vi "Example - Basic IPS-SA.vi"(0 "Connection Details":T6={"VISA resource name"="", "Comms Layer"=enum."Ethernet TCP/IP", "IP Address"="", "Serial Configuration"={"Baud Rate"=115200, "Parity"=0, "Data Bits"=8, "Stop Bits"=10, "Flow Control"=0}, "ISOBUS address"=-1} {"Serial Configuration"."Flow Control" items=["None", "XON/XOFF", "RTS/CTS", "XON/XOFF & RTS/CTS", "DTR/DSR", "XON/XOFF & DTR/DSR"]; "Serial Configuration"."Stop Bits" items=["1.0"=10, "2.0"=20]; "Serial Configuration"."Data Bits" items=["7"=7, "8"=8]; "Serial Configuration"."Parity" items=["None", "Odd", "Even"]; "Serial Configuration"."Baud Rate" items=["300"=300, "600"=600, "1200"=1200, "2400"=2400, "4800"=4800, "9600"=9600, "14400"=14400, "19200"=19200, "38400"=38400, "57600"=57600, "115200"=115200]}, 1 "Axis Group":string(combo)="GRPZ", 2 "ID Query (True)":bool, 3 "Clear Previous Connections (False)":bool, 4 "stop":bool, 6 "Ramp Controls":T8 {"Target Rate (T/min)" format="%_5g"; "Target Field (T)" format="%_5g"; "Target Rate (A/min)" format="%_5g"; "Target Current (A)" format="%_5g"}, 7 "Display Units":bool caption="AMP/TESLA", 8 "Magnet Controls":T9, 9 "SWITCH\nHEATER":bool, 11 "Sw Delay (s)":dbl=30.0 caption="Time Target (s)") -> (10 "System Time":string, 12 "Device Details":T2, 13 "SW HTR\nCONFIRM":bool, 14 "Output Current (A)":dbl format="%.4g", 15 "Magnet Current (A)":dbl format="%.4g", 16 "Output Voltage (V)":dbl format="%.4f", 17 "Current/Field (A/T)":dbl caption="Current Field Factor (A/T)" format="%#.4f", 19 "error out":errorcluster)   [LabVIEW 2013, in "Mercury iXX.lvlib"]
uses:
  Mercury iXX.lvlib
  Public/Libraries/Magnet/Signals/Read/Switch Heater Status (Read).vi
  Public/Libraries/Magnet.lvlib
  Public/Libraries/Magnet/Signals/Read/Current (Read).vi
  Public/Libraries/Magnet/Signals/Read/Persistant Current (Read).vi
  Public/Libraries/Magnet/Configuration/Set/PSU Action Status (Set).vi
  Public/Libraries/Magnet/Controls/PSU Actions.ctl
  Public/Libraries/Magnet/Controls/Switch Heater.ctl
  Public/Libraries/Temperature/Signals/Read/Temperature (Read).vi
  Public/Libraries/Temperature.lvlib
  Public/Libraries/Magnet/Configuration/Read/PSU Action Status (Read).vi
  Public/Libraries/Magnet/Signals/Set/Switch Heater No Check (Set).vi
  Public/Libraries/Magnet/Signals/Set/Target Field (Set).vi
  Public/Libraries/Magnet/Signals/Set/Target Current Rate (Set).vi
  Public/Libraries/Magnet/Signals/Set/Target Current (Set).vi
  Public/Libraries/Magnet/Signals/Set/Target Field Rate (Set).vi
  Public/Libraries/Level Meter/Signals/Read/Probe Level Helium (Read).vi
  Public/Libraries/Level Meter.lvlib
  Public/Libraries/Level Meter/Signals/Read/Probe Level Nitrogen (Read).vi
  Public/Libraries/Magnet/Configuration/Read/PSU Status (Read).vi
  Public/Libraries/System/Read/DateTime (Read).vi
  Public/Libraries/System.lvlib
  Public/Libraries/Pressure/Signals/Read/Current (Read).vi
  Public/Libraries/Pressure.lvlib
  Public/Libraries/System/Open/Open System.vi
  Public/Libraries/System/Read/Catalogue (Read).vi
  Public/Libraries/Level Meter/Open/Open Level Meter Device.vi
  Public/Libraries/Magnet/Open/Open Magnet Device.vi
  Public/Libraries/Magnet/Configuration/Read/Output Configuration (Read).vi
  Public/Libraries/Magnet/Configuration/Read/Current to Field Factor (Read).vi
  Public/Libraries/Temperature/Open/Open Temperature Device.vi
  Public/Libraries/Magnet/Signals/Read/Voltage (Read).vi
  Public/Controls/Comms Transport Layer.ctl
  Public/Controls/Serial Settings.ctl
  Public/Controls/ISOBus Address.ctl
  Public/Libraries/Magnet/Controls/Output Configuration.ctl
panel:
  out "Switch TS":timestamp
  out "Sentinel":bool
  in  "Tab Control":T1(tab)
  in  "Interval between messages (ms)":i16=100
  out "Number of Mag Units\nin the group":dbl
  out "Out Config 2":T7="PARA" caption="Output Configuration"
  out "Sys_time_stamp":timestamp
  out "Mode":string
  out "Nitrogen Level (%)":dbl format="%_4f"
  out "Helium Level (%)":dbl format="%_4f"
  out "Temperature (K)":dbl format="%_4f"
  out "Voltage (V)":dbl(knob) scale=-10.0..10.0
  out "Current (A)":dbl(knob) scale=-60.0..60.0
  out "Elapsed\nTime (s)":dbl caption="Elapsed Time (s)"
  out "Magnet Centre Field (T)":dbl format="%.4f"
  out "Output (T) (Field equivalent)":dbl format="%.4f"
  out "Status":string
  in  "Log file:":string="C:\\temp\\iPS_data.lvm"
  in  "Log Data?":bool
  in  "Plot Data?":bool
  out "Waveform Chart":T10(graph)
  # "Switch Controls"
  # "MercuryiPS-VI"
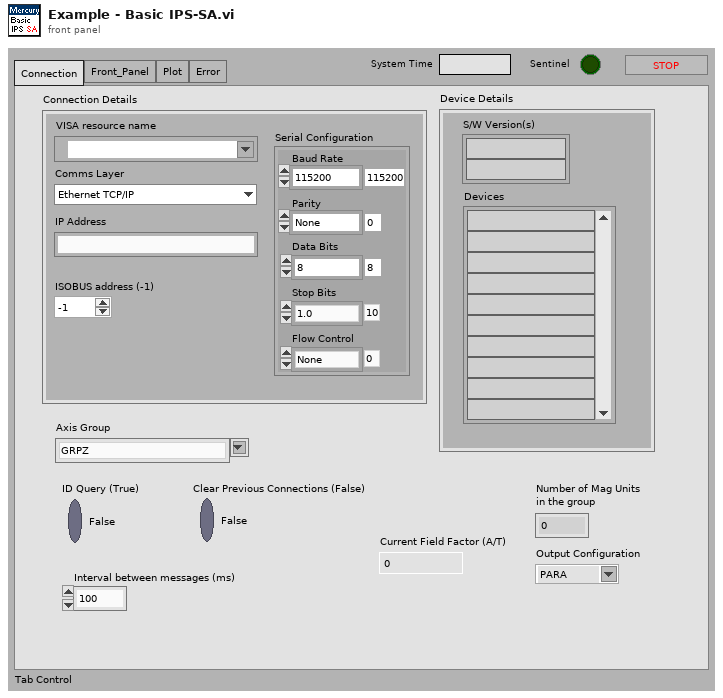
[diagram p1: front panel]
types:
  T1 = enum32{"Connection", "Front_Panel", "Plot", "Error"}
  T2 = cluster{"Devices":string[], "S/W Version(s)":string[]}
  T3 = typedef "Mercury iXX.lvlib/Comms Transport Layer.ctl" = enum16{"Ethernet TCP/IP", "USB", "ISOBus - RS-232", "GPIB"}
  T4 = typedef "Mercury iXX.lvlib/Serial Settings.ctl" = cluster{"Baud Rate":u32, "Parity":u16, "Data Bits":u16, "Stop Bits":u16, "Flow Control":u16}
  T5 = typedef "Mercury iXX.lvlib/ISOBus Address.ctl" = i32
  T6 = cluster{"VISA resource name":refnum<visa-resource-name>, "Comms Layer":T3, "IP Address":string, "Serial Configuration":T4, "ISOBUS address":T5}
  T7 = typedef "Mercury iXX.lvlib/Magnet.lvlib/Output Configuration.ctl" = string
  T8 = cluster{"Target Current (A)":dbl, "Target Rate (A/min)":dbl, "Target Field (T)":dbl, "Target Rate (T/min)":dbl}
  T9 = cluster{"CLAMP":bool, "HOLD":bool, "TO SET":bool, "TO ZERO":bool}
  T10 = cluster{"Current":dbl, "Persistant Current":dbl, "Voltage":dbl, "Temperature":dbl}
  T11 = typedef "Mercury iXX.lvlib/Mercury Reference.ctl" = cluster{"Comms":refnum<visa-resource-name>, "Device ID":string[], "Comms Layer":T3, "Command":string, "Query reference":T12}
  T12 = typedef "Mercury iXX.lvlib/Query Dynamic Reference.ctl" = refnum<vi>
  T13 = typedef "Mercury iXX.lvlib/Magnet.lvlib/PSU Actions.ctl" = string
  T14 = typedef "Mercury iXX.lvlib/Magnet.lvlib/Switch Heater.ctl" = string
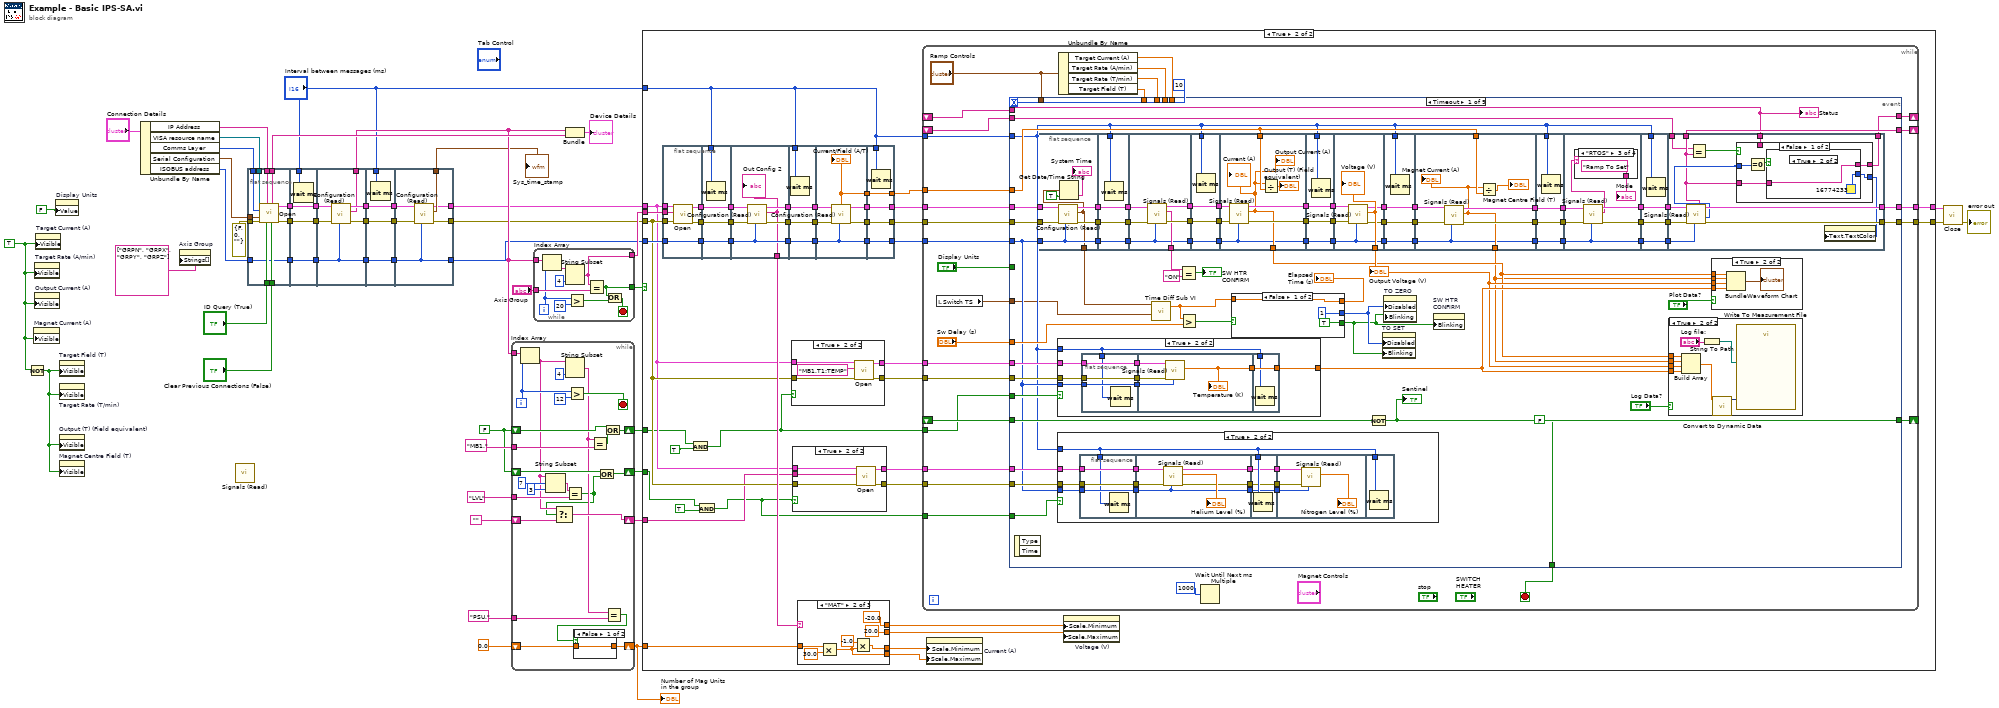
[diagram p0: block diagram]
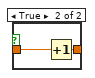
[diagram p2: hidden frame]
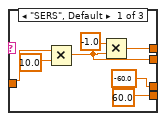
[diagram p6: hidden frame]
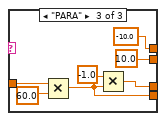
[diagram p7: hidden frame]
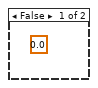
[diagram p8: hidden frame]
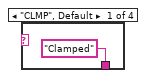
[diagram p9: hidden frame]
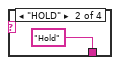
[diagram p10: hidden frame]
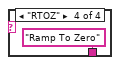
[diagram p11: hidden frame]
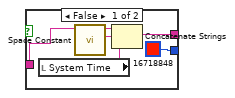
[diagram p12: hidden frame]
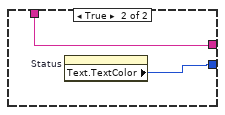
[diagram p13: hidden frame]
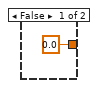
[diagram p14: hidden frame]
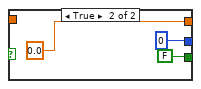
[diagram p17: hidden frame]
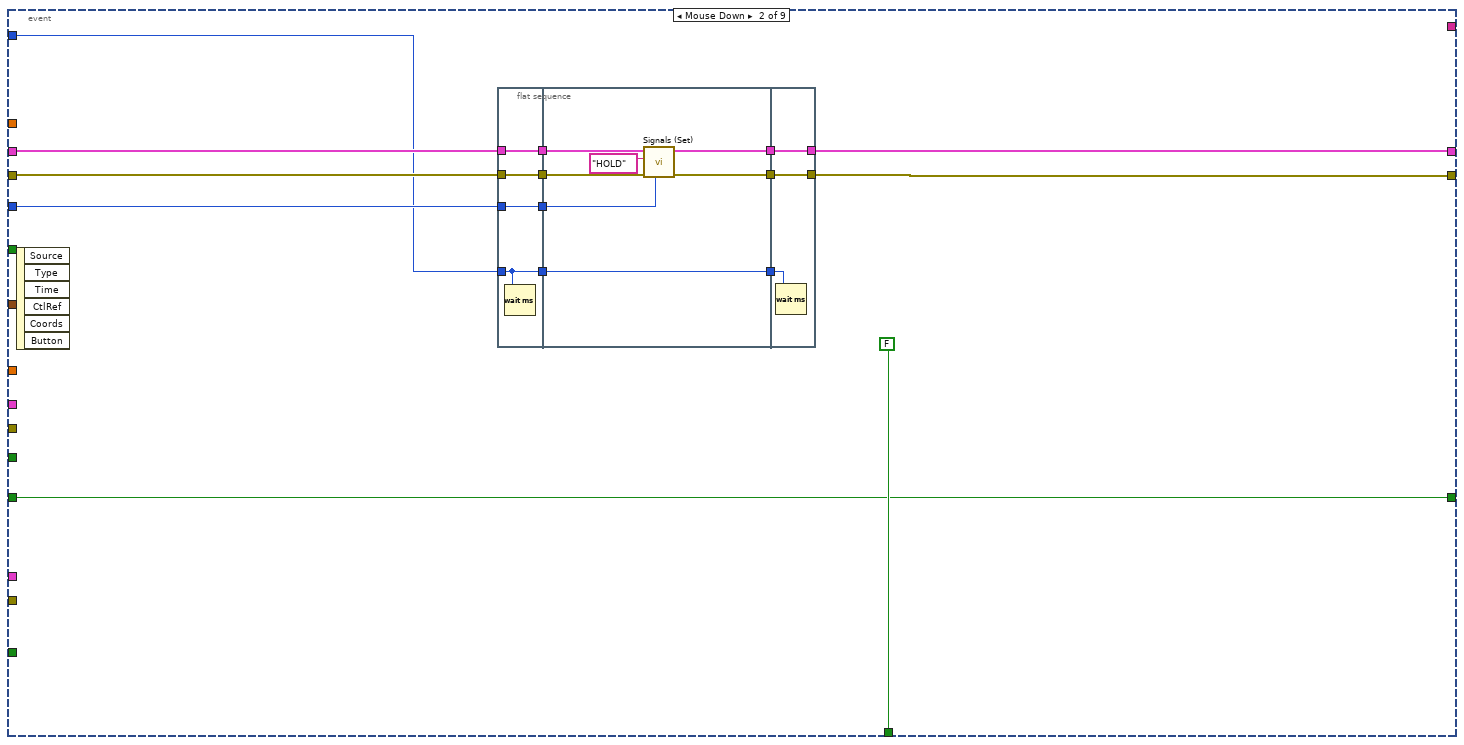
[diagram p18: hidden frame]
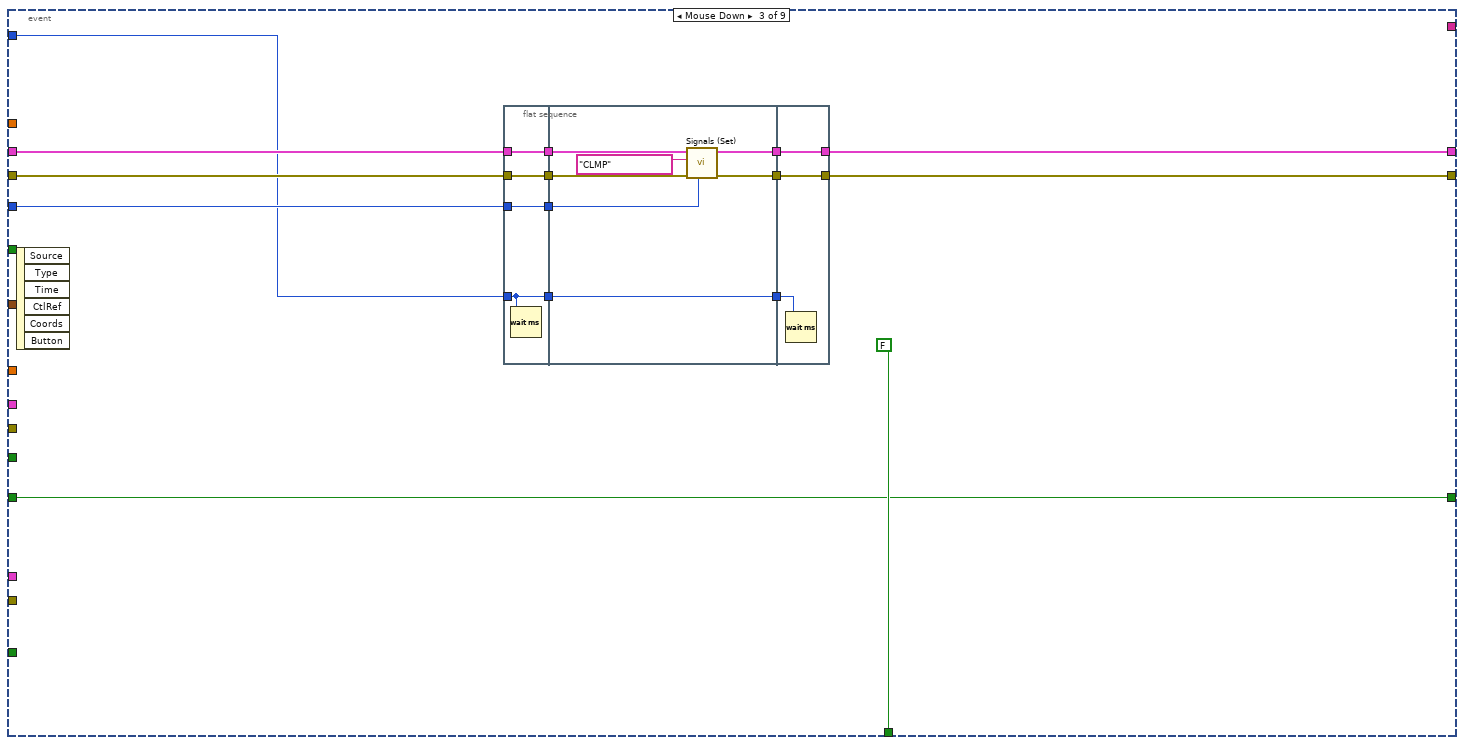
[diagram p19: hidden frame]
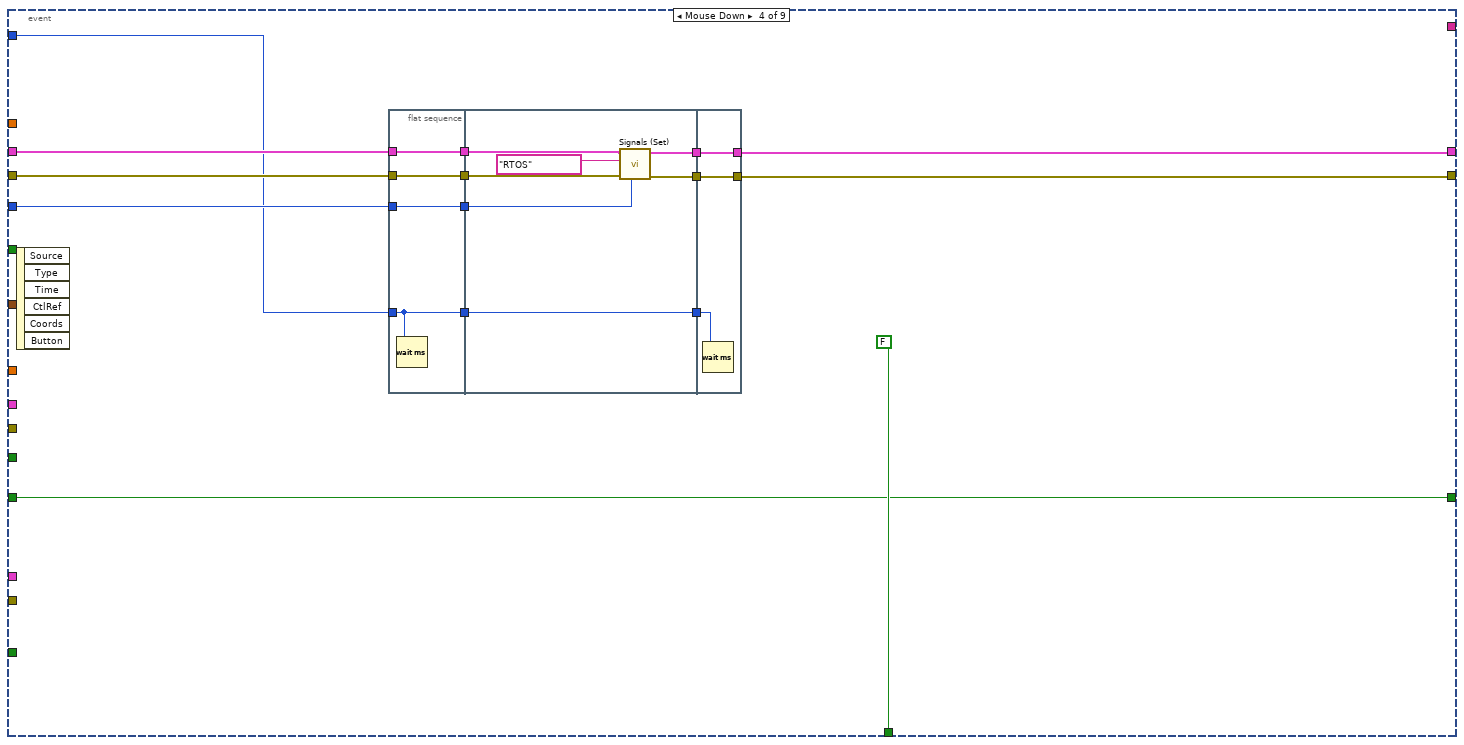
[diagram p20: hidden frame]
diagram:
  w13 = FALSE
  w35 = TRUE ("Visible")
  n1 = Not(x=w35) -> (.not. x?=w34:bool)
  n2 = property on="Magnet Current (A)" class="DigNum (strict)"("Visible"=w35) -> ()  [unwired: 2 in, 2 out]
  n3 = property on="Target Rate (A/min)" class="DigNum (strict)"("Visible"=w35) -> ()  [unwired: 2 in, 2 out]
  n4 = property on="Output Current (A)" class="DigNum (strict)"("Visible"=w35) -> ()  [unwired: 2 in, 2 out]
  n5 = property on="Target Current (A)" class="DigNum (strict)"("Visible"=w35) -> ()  [unwired: 2 in, 2 out]
  n6 = property on="Display Units" class="Bool (strict)"("Value"=FALSE ("AMP/TESLA")) -> ()  [unwired: 2 in, 2 out]
  n7 = property on="Target Field (T)" class="DigNum (strict)"("Visible"=w34) -> ()  [unwired: 2 in, 2 out]
  n8 = property on="Target Rate (T/min)" class="DigNum (strict)"("Visible"=w34) -> ()  [unwired: 2 in, 2 out]
  n9 = property on="Output (T) (Field equivalent)" class="DigNum (strict)"("Visible"=w34) -> ()  [unwired: 2 in, 2 out]
  n10 = property on="Magnet Centre Field (T)" class="DigNum (strict)"("Visible"=w34) -> ()  [unwired: 2 in, 2 out]
  n11 = Unbundle By Name("Connection Details") -> ("IP Address"=w31:string, "VISA resource name"=w30:refnum<visa-resource-name>, "Comms Layer"=w29:T3, "Serial Configuration"=w32:T4, "ISOBUS address"=w20:T5)
  n12 = property on="Axis Group" class="CmbBox"("Strings[]"=string[] ["GRPN", "GRPX", "GRPY", "GRPZ"]) -> ()  [unwired: 2 in, 2 out]
  n13 = call-poly "Signals (Read).vi"() -> ()  [unwired: 7 in, 5 out]
  n14 = flat-sequence {
    tunnel: errorcluster {"status"=FALSE, "code"=0, "source"=""} ("error in (no error)") -> [w60]
    tunnel: "ID Query (True)" -> [w59]
    tunnel: "Clear Previous Connections (False)" -> [w58]
    tunnel: w32 -> [w55]
    tunnel: w31 -> [w54]
    tunnel: w30 -> [w53]
    tunnel: w29 -> [w52]
    tunnel: [w51] -> w27
    tunnel: [w57] -> w24
    tunnel: [w56] -> w23
    tunnel: w20 -> [w50]
    tunnel: [w50] -> w19
    tunnel: w24 -> [w64]
    tunnel: w23 -> [w63]
    tunnel: [w64] -> w22
    tunnel: [w63] -> w21
    tunnel: w19 -> [w62]
    tunnel: [w62] -> w18
    tunnel: "Interval between messages (ms)" -> [w61]
    tunnel: w22 -> [w69]
    tunnel: w21 -> [w68]
    tunnel: w18 -> [w70]
    tunnel: [w70] -> w17
    tunnel: [w67] -> w16
    tunnel: [w66] -> w15
    tunnel: [w65] -> w6
    tunnel: w17 -> [w74]
    tunnel: w16 -> [w73]
    tunnel: w15 -> [w72]
    tunnel: "Interval between messages (ms)" -> [w71]
    tunnel: [w74] -> w9
    tunnel: [w73] -> w8
    tunnel: [w72] -> w7
    tunnel: w9 -> [w78]
    tunnel: w8 -> [w79]
    tunnel: w7 -> [w80]
    tunnel: [w77] -> w1
    tunnel: [w78] -> w5
    tunnel: [w76] -> w3
    tunnel: [w75] -> w2
    frame #0 {
      n15 = call-poly "Open.vi"("Clear Previous Connections (False)"=w58, "ID Query (True)"=w59, "IP Address"=w54, "error in (no error)"=w60, "Serial Configuration"=w55, "Comms Layer"=w52, "VISA resource name"=w53) -> ("error out"=w56:errorcluster, "Mercury Reference Out"=w57:T11, "S/W Version(s)"=w51:string[])  [unwired: 2 out]
    }
    frame #1 {
      n16 = Wait (ms)(milliseconds to wait=w61) -> ()  [unwired: 1 out]
    }
    frame #2 {
      n17 = call-poly "Configuration (Read).vi"("ISOBUS address"=w70, "error in"=w68, "Mercury Reference In"=w69) -> ("error out"=w67:errorcluster, "Devices"=w65:string[], "Mercury Reference Out"=w66:T11)  [unwired: 6 out]
    }
    frame #3 {
      n18 = Wait (ms)(milliseconds to wait=w71) -> ()  [unwired: 1 out]
    }
    frame #4 {
      n19 = call-poly "Configuration (Read).vi"("ISOBUS address"=w78, "error in"=w79, "Mercury Reference In"=w80) -> ("error out"=w75:errorcluster, "time stamp"=w77:timestamp, "Mercury Reference Out"=w76:T11)  [unwired: 6 out]
    }
  }
  n20 = while {
    shift-right: [w101] -> w37
    shift-left: 0.0 -> [w100]
    tunnel: "PSU." -> [w97]
    tunnel: w6 -> [w96]
    shift-right: [w93] -> w25
    shift-left: w13 -> [w92]
    tunnel: "MB1." -> [w94]
    tunnel: "LVL" -> [w88]
    shift-right: [w86] -> w12
    shift-left: w13 -> [w87]
    shift-right: [w84] -> w10
    shift-left: "" -> [w85]
    i -> [w102]
    stop <- w98 stop-if-true
    n21 = Index Array(array=w96, index=w102) -> (element=w82:string)
    n22 = String Subset(string=w82, offset (0)=7, length (rest)=3 ("length (rest)")) -> (substring=w89:string)
    n23 = String Subset(string=w82, length (rest)=4 ("length (rest)")) -> (substring=w83:string)  [unwired: 1 out]
    n24 = Equal?(x=w89, y=w88) -> (x = y?=w81:bool)
    n25 = Select(t=w82, s=w81, f=w85) -> (s? t:f=w84:string)
    n26 = Greater?(x=w102, y=12) -> (0:w98:bool)
    n27 = Equal?(x=w83, y=w94) -> (x = y?=w95:bool)
    n28 = Or(x=w87, y=w81) -> (x .or. y?=w86:bool)
    n29 = Or(x=w92, y=w95) -> (x .or. y?=w93:bool)
    n30 = Equal?(x=w83, y=w97) -> (x = y?=w99:bool)
    n31 = case shown="False" w99 {
      tunnel: [w105 w107] -> w101
      tunnel: w100 -> [w105 w106]
      frame False {
      }
      frame True {
        n32 = Increment(x=w106) -> (x+1=w107:dbl)
      }
    }
  }
  "Number of Mag Units\nin the group" <- w37
  n33 = while {
    tunnel: w6 -> [w117]
    tunnel: [w108] -> w45
    tunnel: "Axis Group" -> [w114]
    tunnel: [w109] -> w46
    i -> [w112]
    stop <- w111 stop-if-true
    n34 = Index Array(array=w117, index=w112) -> (element=w115:string)
    n35 = String Subset(string=w115, length (rest)=4 ("length (rest)")) -> (substring=w108:string)  [unwired: 1 out]
    n36 = Greater?(x=w112, y=20) -> (0:w110:bool)
    n37 = Equal?(x=w108, y=w114) -> (x = y?=w109:bool)
    n38 = Or(x=w109, y=w110) -> (x .or. y?=w111:bool)
  }
  n39 = Bundle("Devices"=w6, "S/W Version(s)"=w27) -> (→"Device Details":T2)  [unwired: 1 out]
  n40 = case shown="True" w46 {
    tunnel: w3 -> [w119 w129]
    tunnel: w45 -> [_ w163]
    tunnel: w5 -> [_ w153]
    tunnel: [w119 w162] -> w44
    tunnel: [w118 w161] -> w43
    tunnel: w37 -> [_ w160]
    tunnel: w2 -> [w118 w130]
    tunnel: w25 -> [_ w125]
    tunnel: "Interval between messages (ms)" -> [_ w131]
    tunnel: w12 -> [_ w123]
    tunnel: w10 -> [_ w128]
    frame False {
    }
    frame True {
      n41 = flat-sequence {
        tunnel: w163 -> [w176]
        tunnel: w130 -> [w173]
        tunnel: w129 -> [w172]
        tunnel: w153 -> [w171]
        tunnel: [w175] -> w152
        tunnel: [w174] -> w151
        tunnel: [w171] -> w150
        tunnel: w152 -> [w180]
        tunnel: w151 -> [w179]
        tunnel: w150 -> [w178]
        tunnel: [w180] -> w149
        tunnel: [w179] -> w148
        tunnel: [w178] -> w147
        tunnel: w131 -> [w177]
        tunnel: w149 -> [w186]
        tunnel: w148 -> [w185]
        tunnel: w147 -> [w184]
        tunnel: [w181] -> w146
        tunnel: [w184] -> w145
        tunnel: [w183] -> w144
        tunnel: [w182] -> w143
        tunnel: w145 -> [w190]
        tunnel: w144 -> [w189]
        tunnel: w143 -> [w188]
        tunnel: [w190] -> w142
        tunnel: [w189] -> w141
        tunnel: [w188] -> w140
        tunnel: w131 -> [w187]
        tunnel: w142 -> [w192]
        tunnel: w141 -> [w196]
        tunnel: w140 -> [w195]
        tunnel: [w192] -> w139
        tunnel: [w194] -> w138
        tunnel: [w193] -> w137
        tunnel: [w191] -> w136
        tunnel: [w198] -> w135
        tunnel: [w199] -> w133
        tunnel: [w200] -> w134
        tunnel: [w201] -> w132
        tunnel: w139 -> [w201]
        tunnel: w138 -> [w200]
        tunnel: w137 -> [w199]
        tunnel: w136 -> [w198]
        tunnel: w131 -> [w197]
        frame #0 {
          n42 = call-poly "Open.vi"("error in (no error)"=w173, "Device Identifier"=w176, "Mercury Reference In"=w172) -> ("error out"=w174:errorcluster, "Mercury Reference Out"=w175:T11)  [unwired: 7 out]
        }
        frame #1 {
          n43 = Wait (ms)(milliseconds to wait=w177) -> ()  [unwired: 1 out]
        }
        frame #2 {
          n44 = call-poly "Configuration (Read).vi"("ISOBUS address"=w184, "error in"=w185, "Mercury Reference In"=w186) -> ("error out"=w182:errorcluster, "Out Config"=w181:T7, "Mercury Reference Out"=w183:T11)  [unwired: 6 out]
          "Out Config 2" <- w181
        }
        frame #3 {
          n45 = Wait (ms)(milliseconds to wait=w187) -> ()  [unwired: 1 out]
        }
        frame #4 {
          n46 = call-poly "Configuration (Read).vi"("ISOBUS address"=w192, "error in"=w195, "Mercury Reference In"=w196) -> ("error out"=w193:errorcluster, "AtoB"=w191:dbl, "Mercury Reference Out"=w194:T11)  [unwired: 6 out]
          "Current/Field (A/T)" <- w191
        }
        frame #5 {
          n47 = Wait (ms)(milliseconds to wait=w197) -> ()  [unwired: 1 out]
        }
      }
      n48 = And(x=w125, y=TRUE) -> (x .and. y?=w124:bool)
      n49 = And(x=w123, y=TRUE) -> (x .and. y?=w122:bool)
      n50 = case shown="True" w124 {
        tunnel: w130 -> [w202 w207]
        tunnel: w129 -> [w203 w206]
        tunnel: [w203 w205] -> w155
        tunnel: [w202 w204] -> w154
        frame False {
        }
        frame True {
          n51 = call-poly "Open.vi"("error in (no error)"=w207, "Device Identifier"="MB1.T1:TEMP", "Mercury Reference In"=w206) -> ("error out"=w204:errorcluster, "Mercury Reference Out"=w205:T11)  [unwired: 7 out]
        }
      }
      n52 = case shown="True" w122 {
        tunnel: w130 -> [w164 w170]
        tunnel: w129 -> [w165 w169]
        tunnel: [w165 w168] -> w127
        tunnel: [w164 w167] -> w126
        tunnel: w128 -> [_ w166]
        frame False {
        }
        frame True {
          n53 = call-poly "Open.vi"("error in (no error)"=w170, "Device Identifier"=w166, "Mercury Reference In"=w169) -> ("error out"=w167:errorcluster, "Mercury Reference Out"=w168:T11)  [unwired: 7 out]
        }
      }
      n54 = case shown="\"MAT\"" w146 {
        tunnel: w160 -> [w213 w220 w229]
        tunnel: [60.0 ("y") w219 w226] -> w158
        tunnel: [-60.0 ("y") w218 w225] -> w159
        tunnel: [w212 -20.0 ("y") -10.0 ("y")] -> w157
        tunnel: [w211 20.0 ("y") 10.0 ("y")] -> w156
        frame "SERS", Default {
          n55 = Multiply(x=w213, y=10.0) -> (x*y=w211:dbl)
          n56 = Multiply(x=-1.0, y=w211) -> (x*y=w212:dbl)
        }
        frame "MAT" {
          n57 = Multiply(x=w220, y=30.0) -> (x*y=w219:dbl)
          n58 = Multiply(x=-1.0, y=w219) -> (x*y=w218:dbl)
        }
        frame "PARA" {
          n59 = Multiply(x=w229, y=60.0) -> (x*y=w226:dbl)
          n60 = Multiply(x=-1.0, y=w226) -> (x*y=w225:dbl)
        }
      }
      n61 = while {
        tunnel: w134 -> [w257]
        tunnel: w133 -> [w256]
        shift-right: [w254] -> _
        shift-left: _ -> [w255]
        tunnel: [w252] -> w162
        tunnel: [w251] -> w161
        tunnel: w135 -> [w249]
        tunnel: w155 -> [w242]
        tunnel: w154 -> [w241]
        tunnel: w124 -> [w243]
        tunnel: w132 -> [w240]
        tunnel: w131 -> [w239]
        tunnel: w127 -> [w238]
        tunnel: w126 -> [w237]
        tunnel: w122 -> [w236]
        shift-right: [w235] -> _
        shift-left: _ -> [w234]
        shift-right: [w233] -> _
        shift-left: _ -> [w232]
        stop <- w253 stop-if-true
        n62 = local read "Switch TS"() -> (w231:timestamp)
        n63 = Unbundle By Name("Ramp Controls") -> ("Target Current (A)"=w246:dbl, "Target Rate (A/min)"=w247:dbl, "Target Rate (T/min)"=w245:dbl, "Target Field (T)"=w244:dbl)
        n64 = event shown="[0] Timeout" {
          selector: _ -> [_ _ _ _ _ _ _ _ _]
          dyn-events: _ -> [_ _ _ _ _ _ _ _ _]
          timeout: 10 -> [_ _ _ _ _ _ _ _ _]
          tunnel: w257 -> [w316 w514 w544 w573 w602 w639 w754 w874 w877]
          tunnel: w256 -> [w315 w515 w543 w572 w601 w638 w753 w873 w888]
          tunnel: w255 -> [w330 w510 w539 w568 w597 w643 w749 w875 _]
          tunnel: [w329 w510 w539 w568 w597 w643 w749 w875 _] -> w254
          tunnel: [w290 w513 w542 w571 w600 w642 w752 w874 w877] -> w252
          tunnel: [w289 w512 w541 w570 w599 w641 w751 w873 w880] -> w251
          tunnel: [FALSE FALSE FALSE FALSE FALSE FALSE FALSE TRUE _] -> w253
          tunnel: "Sw Delay (s)" -> [w327 _ _ _ _ _ _ _ _]
          tunnel: w249 -> [w278 _ _ _ _ _ w740 _ _]
          tunnel: "Display Units" -> [_ _ _ _ _ _ w748 _ w879]
          tunnel: w247 -> [_ _ _ _ _ _ w747 _ _]
          tunnel: w246 -> [_ _ _ _ _ _ w746 _ _]
          tunnel: w245 -> [_ _ _ _ _ _ w745 _ _]
          tunnel: w244 -> [_ _ _ _ _ _ w744 _ _]
          tunnel: w243 -> [w320 _ _ _ _ _ _ _ _]
          tunnel: w242 -> [w319 _ _ _ _ _ _ _ _]
          tunnel: w241 -> [w318 _ _ _ _ _ _ _ _]
          tunnel: w240 -> [w273 w509 w538 w567 w596 w637 w743 _ _]
          tunnel: w239 -> [w272 w501 w530 w559 w588 w617 w742 _ _]
          tunnel: w238 -> [w275 _ _ _ _ _ _ _ _]
          tunnel: w237 -> [w274 _ _ _ _ _ _ _ _]
          tunnel: w236 -> [w271 _ _ _ _ _ _ _ _]
          tunnel: [w266 _ _ _ _ _ _ _ _] -> w235
          tunnel: w234 -> [w265 _ _ _ _ _ _ _ _]
          tunnel: [w264 _ _ _ _ _ _ _ _] -> w233
          tunnel: w232 -> [w260 _ _ _ _ _ _ _ _]
          tunnel: w231 -> [w262 _ _ _ _ _ _ _ _]
          tunnel: "Ramp Controls" -> [_ _ _ _ _ _ w741 _ _]
          event Timeout {
            n65 = event-data() -> ()  [unwired: 3 out]
            n66 = flat-sequence {
              tunnel: [w367] -> w263
              tunnel: w316 -> [w372]
              tunnel: w315 -> [w371]
              tunnel: [w370] -> w314
              tunnel: [w369] -> w313
              tunnel: w273 -> [w368]
              tunnel: [w368] -> w287
              tunnel: w314 -> [w376]
              tunnel: w313 -> [w375]
              tunnel: [w376] -> w312
              tunnel: [w375] -> w311
              tunnel: [w374] -> w288
              tunnel: w287 -> [w374]
              tunnel: w272 -> [w373]
              tunnel: w312 -> [w381]
              tunnel: w311 -> [w382]
              tunnel: [w378] -> w310
              tunnel: [w380] -> w309
              tunnel: [w379] -> w308
              tunnel: w288 -> [w377]
              tunnel: [w377] -> w285
              tunnel: w309 -> [w386]
              tunnel: w308 -> [w385]
              tunnel: [w386] -> w307
              tunnel: [w385] -> w306
              tunnel: [w384] -> w286
              tunnel: w285 -> [w384]
              tunnel: w272 -> [w383]
              tunnel: w307 -> [w394]
              tunnel: w306 -> [w393]
              tunnel: w278 -> [w391]
              tunnel: [w390] -> w305
              tunnel: [w389] -> w304
              tunnel: [w388] -> w300
              tunnel: w286 -> [w387]
              tunnel: [w387] -> w283
              tunnel: w305 -> [w398]
              tunnel: w304 -> [w397]
              tunnel: [w398] -> w303
              tunnel: [w397] -> w302
              tunnel: [w396] -> w284
              tunnel: w283 -> [w396]
              tunnel: w272 -> [w395]
              tunnel: w303 -> [w404]
              tunnel: w302 -> [w403]
              tunnel: [w402] -> w301
              tunnel: [w401] -> w299
              tunnel: [w400] -> w298
              tunnel: w284 -> [w399]
              tunnel: [w399] -> w281
              tunnel: w299 -> [w408]
              tunnel: w298 -> [w407]
              tunnel: [w408] -> w297
              tunnel: [w407] -> w296
              tunnel: [w406] -> w282
              tunnel: w281 -> [w406]
              tunnel: w272 -> [w405]
              tunnel: w297 -> [w416]
              tunnel: w296 -> [w415]
              tunnel: w278 -> [w411]
              tunnel: [w410] -> w295
              tunnel: [w414] -> w294
              tunnel: [w413] -> w293
              tunnel: w282 -> [w409]
              tunnel: [w409] -> w279
              tunnel: w294 -> [w420]
              tunnel: w293 -> [w419]
              tunnel: [w420] -> w292
              tunnel: [w419] -> w291
              tunnel: [w418] -> w280
              tunnel: w279 -> [w418]
              tunnel: w272 -> [w417]
              tunnel: w292 -> [w426]
              tunnel: w291 -> [w427]
              tunnel: w280 -> [w423]
              tunnel: [w425] -> w277
              tunnel: [w424] -> w276
              tunnel: [w423] -> w267
              tunnel: w277 -> [w435]
              tunnel: w276 -> [w434]
              tunnel: w272 -> [w433]
              tunnel: [w435] -> w270
              tunnel: [w434] -> w269
              tunnel: [w432] -> w268
              tunnel: w267 -> [w432]
              tunnel: [w444] -> w289
              tunnel: [w445] -> w290
              tunnel: w270 -> [w446]
              tunnel: w269 -> [w447]
              tunnel: w268 -> [w443]
              tunnel: [w439] -> w266
              tunnel: w265 -> [w438]
              tunnel: [w437] -> w264
              tunnel: w260 -> [w436]
              frame #0 {
                n67 = call-poly "Configuration (Read).vi"("ISOBUS address"=w368, "error in"=w371, "Mercury Reference In"=w372) -> ("error out"=w369:errorcluster, "time stamp"=w367:timestamp, "Mercury Reference Out"=w370:T11)  [unwired: 6 out]
                n68 = Get Date/Time String(seconds (now)=w367, want seconds? (F)=TRUE) -> (time string=→"System Time":string)  [unwired: 1 in, 1 out]
              }
              frame #1 {
                n69 = Wait (ms)(milliseconds to wait=w373) -> ()  [unwired: 1 out]
              }
              frame #2 {
                n70 = call-poly "Signals (Read).vi"("ISOBUS address"=w377, "error in"=w382, "Mercury Reference In"=w381) -> ("error out"=w379:errorcluster, "Switch Heater Status"=w378:string, "Mercury Reference Out"=w380:T11)  [unwired: 6 out]
              }
              frame #3 {
                n71 = Wait (ms)(milliseconds to wait=w383) -> ()  [unwired: 1 out]
              }
              frame #4 {
                n72 = call-poly "Signals (Read).vi"("ISOBUS address"=w387, "error in"=w393, "Mercury Reference In"=w394) -> ("error out"=w389:errorcluster, "Current"=w388:dbl, "Mercury Reference Out"=w390:T11)  [unwired: 6 out]
                "Current (A)" <- w388
                "Output Current (A)" <- w388
                n73 = Divide(x=w388, y=w391) -> (x/y=→"Output (T) (Field equivalent)":dbl)
              }
              frame #5 {
                n74 = Wait (ms)(milliseconds to wait=w395) -> ()  [unwired: 1 out]
              }
              frame #6 {
                n75 = call-poly "Signals (Read).vi"("ISOBUS address"=w399, "error in"=w403, "Mercury Reference In"=w404) -> ("error out"=w400:errorcluster, "Voltage"=w402:dbl, "Mercury Reference Out"=w401:T11)  [unwired: 6 out]
                "Voltage (V)" <- w402
              }
              frame #7 {
                n76 = Wait (ms)(milliseconds to wait=w405) -> ()  [unwired: 1 out]
              }
              frame #8 {
                n77 = call-poly "Signals (Read).vi"("ISOBUS address"=w409, "error in"=w415, "Mercury Reference In"=w416) -> ("error out"=w414:errorcluster, "Persistant Current"=w410:dbl, "Mercury Reference Out"=w413:T11)  [unwired: 6 out]
                "Magnet Current (A)" <- w410
                n78 = Divide(x=w410, y=w411) -> (x/y=→"Magnet Centre Field (T)":dbl)
              }
              frame #9 {
                n79 = Wait (ms)(milliseconds to wait=w417) -> ()  [unwired: 1 out]
              }
              frame #10 {
                n80 = call-poly "Signals (Read).vi"("ISOBUS address"=w423, "error in"=w426, "Mercury Reference In"=w427) -> ("error out"=w424:errorcluster, "PSU Act Stat"=w422:T13, "Mercury Reference Out"=w425:T11)  [unwired: 6 out]
                n81 = case shown="\"RTOS\"" w422 {
                  tunnel: ["Clamped" "Hold" "Ramp To Set" "Ramp To Zero"] -> w421
                  frame "CLMP", Default {
                  }
                  frame "HOLD" {
                  }
                  frame "RTOS" {
                  }
                  frame "RTOZ" {
                  }
                }
                "Mode" <- w421
              }
              frame #11 {
                n82 = Wait (ms)(milliseconds to wait=w433) -> ()  [unwired: 1 out]
              }
              frame #12 {
                n83 = call-poly "Signals (Read).vi"("ISOBUS address"=w443, "error in"=w447, "Mercury Reference In"=w446) -> ("error out"=w444:errorcluster, "Status Hex value"=w442:i32, "Mercury Reference Out"=w445:T11, "Status"=w439:string)  [unwired: 3 in, 2 out]
                n84 = Equal?(x=w438, y=w439) -> (x = y?=w440:bool)
                n85 = case shown="False" w440 {
                  tunnel: w442 -> [w452 _]
                  tunnel: w439 -> [w451 _]
                  tunnel: [w449 w461] -> w437
                  tunnel: [w448 w460] -> w441
                  tunnel: w436 -> [_ w461]
                  frame False {
                    n86 = Equal To 0?(x=w452) -> (x = 0?=w450:bool)
                    n87 = case shown="True" w450 {
                      tunnel: w451 -> [w454 w458]
                      tunnel: [w453 w458] -> w449
                      tunnel: [u32 16718848 ("Text.Text Colors:Text Color") u32 16774233 ("Text.Text Colors:Text Color")] -> w448
                      frame False {
                        n88 = local read "System Time"() -> (w456:string)
                        n89 = call <vilib>:"Space Constant.vi"() -> ("String"=w455:string)
                        n90 = Concatenate Strings(w454, w455, w456) -> (w453:string)
                      }
                      frame True {
                      }
                    }
                  }
                  frame True {
                    n91 = property on="Status" class="Str"() -> ("Text.TextColor"=w460:u32)  [unwired: 2 in, 2 out]
                  }
                }
                n92 = property on="Status" class="Str"("Text.TextColor"=w441) -> ()  [unwired: 2 in, 2 out]
              }
            }
            n93 = case shown="True" w320 {
              tunnel: w319 -> [_ w471]
              tunnel: w318 -> [_ w470]
              tunnel: [0.0 ("Temperature") w469] -> w317
              tunnel: w273 -> [_ w468]
              tunnel: w272 -> [_ w463]
              frame False {
              }
              frame True {
                n94 = flat-sequence {
                  tunnel: w468 -> [w473]
                  tunnel: w470 -> [w474]
                  tunnel: w471 -> [w475]
                  tunnel: [w475] -> w466
                  tunnel: [w474] -> w465
                  tunnel: [w473] -> w464
                  tunnel: w463 -> [w472]
                  tunnel: [w477] -> w467
                  tunnel: w466 -> [w479]
                  tunnel: w465 -> [w478]
                  tunnel: w464 -> [w476]
                  tunnel: [w481] -> w469
                  tunnel: w467 -> [w481]
                  tunnel: w463 -> [w480]
                  frame #0 {
                    n95 = Wait (ms)(milliseconds to wait=w472) -> ()  [unwired: 1 out]
                  }
                  frame #1 {
                    n96 = call-poly "Signals (Read).vi"("ISOBUS address"=w476, "error in"=w478, "Mercury Reference In"=w479) -> ("Temperature"=w477:dbl)  [unwired: 4 in, 4 out]
                    "Temperature (K)" <- w477
                  }
                  frame #2 {
                    n97 = Wait (ms)(milliseconds to wait=w480) -> ()  [unwired: 1 out]
                  }
                }
              }
            }
            n98 = case shown="True" w271 {
              tunnel: w275 -> [_ w345]
              tunnel: w274 -> [_ w344]
              tunnel: w273 -> [_ w343]
              tunnel: w272 -> [_ w333]
              frame False {
                (unwired) 0.0 ("Temperature")
              }
              frame True {
                n99 = flat-sequence {
                  tunnel: w343 -> [w347]
                  tunnel: w344 -> [w348]
                  tunnel: w345 -> [w349]
                  tunnel: [w349] -> w342
                  tunnel: [w348] -> w341
                  tunnel: [w347] -> w340
                  tunnel: w333 -> [w346]
                  tunnel: w342 -> [w355]
                  tunnel: w341 -> [w354]
                  tunnel: w340 -> [w350]
                  tunnel: [w352] -> w338
                  tunnel: [w351] -> w336
                  tunnel: [w350] -> w334
                  tunnel: w333 -> [w359]
                  tunnel: [w358] -> w339
                  tunnel: w338 -> [w358]
                  tunnel: [w357] -> w337
                  tunnel: w336 -> [w357]
                  tunnel: [w356] -> w335
                  tunnel: w334 -> [w356]
                  tunnel: w339 -> [w363]
                  tunnel: w337 -> [w362]
                  tunnel: w335 -> [w361]
                  tunnel: w333 -> [w364]
                  frame #0 {
                    n100 = Wait (ms)(milliseconds to wait=w346) -> ()  [unwired: 1 out]
                  }
                  frame #1 {
                    n101 = call-poly "Signals (Read).vi"("ISOBUS address"=w350, "error in"=w354, "Mercury Reference In"=w355) -> ("error out"=w351:errorcluster, "Level"=→"Helium Level (%)":dbl, "Mercury Reference Out"=w352:T11)  [unwired: 4 in, 2 out]
                  }
                  frame #2 {
                    n102 = Wait (ms)(milliseconds to wait=w359) -> ()  [unwired: 1 out]
                  }
                  frame #3 {
                    n103 = call-poly "Signals (Read).vi"("ISOBUS address"=w361, "error in"=w362, "Mercury Reference In"=w363) -> ("Level"=→"Nitrogen Level (%)":dbl)  [unwired: 4 in, 4 out]
                  }
                  frame #4 {
                    n104 = Wait (ms)(milliseconds to wait=w364) -> ()  [unwired: 1 out]
                  }
                }
              }
            }
            n105 = call "Time Diff Sub VI.vi"("Start Time Stamp"=w262, "Current Time Stamp"=w263) -> ("Time Diff"=w261:dbl)  [unwired: 2 in, 1 out]
            n106 = Equal?(x=w310, y="ON") -> (x = y?=→"SW HTR\nCONFIRM":bool)
            n107 = Greater?(x=w261, y=w327) -> (0:w326:bool)
            n108 = case shown="False" w326 {
              tunnel: [w497 0.0 ("Elapsed\nTime (s)")] -> w325
              tunnel: w261 -> [w497 _]
              tunnel: [TRUE ("Blinking") FALSE ("Blinking")] -> w323
              tunnel: [u8 1 ("Disabled") u8 0 ("Disabled")] -> w324
              frame False {
              }
              frame True {
              }
            }
            "Elapsed\nTime (s)" <- w325
            n109 = Not(x=w330) -> (.not. x?=w329:bool)
            "Sentinel" <- w329
            n110 = property on="TO SET" class="Bool"("Disabled"=w324, "Blinking"=w323) -> ()  [unwired: 2 in, 2 out]
            n111 = property on="TO ZERO" class="Bool"("Disabled"=w324, "Blinking"=w323) -> ()  [unwired: 2 in, 2 out]
            n112 = property on="SW HTR\nCONFIRM" class="Bool (strict)"("Blinking"=w323) -> ()  [unwired: 2 in, 2 out]
            n113 = case shown="True" "Log Data?" {
              tunnel: w301 -> [_ w487]
              tunnel: w317 -> [_ w484]
              tunnel: w300 -> [_ w483]
              tunnel: w295 -> [_ w482]
              frame False {
              }
              frame True {
                n114 = Build Array(w483, w482, w487, w484) -> (w486:dbl[])
                n115 = String To Path(string="Log file:") -> (path=w488:path)
                n116 = call "Convert to Dynamic Data"("Array"=w486) -> ("Dynamic Data Type"=w485:dynamicdata)  [unwired: 3 in]
                n117 = call "Write To Measurement File"("Signals"=w485, "Filename"=w488) -> ()  [unwired: 15 in, 3 out]
              }
            }
            n118 = case shown="True" "Plot Data?" {
              tunnel: w301 -> [_ w494]
              tunnel: w317 -> [_ w493]
              tunnel: w300 -> [_ w492]
              tunnel: w295 -> [_ w491]
              frame False {
              }
              frame True {
                n119 = Bundle("Current"=w492, "Persistant Current"=w491, "Voltage"=w494, "Temperature"=w493) -> (→"Waveform Chart":T10)  [unwired: 1 in]
              }
            }
            "Output Voltage (V)" <- w301
            "Status" <- w260
          }
          event "Magnet Controls.HOLD": Mouse Down {
            n120 = event-data() -> ()  [unwired: 7 out]
            n121 = flat-sequence {
              tunnel: w509 -> [w517]
              tunnel: w514 -> [w518]
              tunnel: w515 -> [w519]
              tunnel: [w519] -> w508
              tunnel: [w518] -> w507
              tunnel: [w517] -> w506
              tunnel: [w516] -> w502
              tunnel: w501 -> [w516]
              tunnel: w508 -> [w526]
              tunnel: w507 -> [w525]
              tunnel: w506 -> [w521]
              tunnel: [w524] -> w505
              tunnel: [w523] -> w504
              tunnel: [w520] -> w503
              tunnel: w502 -> [w520]
              tunnel: [w528] -> w512
              tunnel: [w529] -> w513
              tunnel: w505 -> [w529]
              tunnel: w504 -> [w528]
              tunnel: w503 -> [w527]
              frame #0 {
                n122 = Wait (ms)(milliseconds to wait=w516) -> ()  [unwired: 1 out]
              }
              frame #1 {
                n123 = call-poly "Signals (Set).vi"("ISOBUS address"=w521, "error in"=w526, "PSU Act Stat"=T13 "HOLD", "Mercury Reference In"=w525) -> ("error out"=w523:errorcluster, "Mercury Reference Out"=w524:T11)  [unwired: 6 out]
              }
              frame #2 {
                n124 = Wait (ms)(milliseconds to wait=w527) -> ()  [unwired: 1 out]
              }
            }
          }
          event "Magnet Controls.CLAMP": Mouse Down {
            n125 = event-data() -> ()  [unwired: 7 out]
            n126 = flat-sequence {
              tunnel: w538 -> [w546]
              tunnel: w543 -> [w547]
              tunnel: w544 -> [w548]
              tunnel: [w548] -> w537
              tunnel: [w547] -> w536
              tunnel: [w546] -> w535
              tunnel: [w545] -> w531
              tunnel: w530 -> [w545]
              tunnel: w537 -> [w555]
              tunnel: w536 -> [w554]
              tunnel: w535 -> [w550]
              tunnel: [w553] -> w534
              tunnel: [w552] -> w533
              tunnel: [w549] -> w532
              tunnel: w531 -> [w549]
              tunnel: [w557] -> w541
              tunnel: [w558] -> w542
              tunnel: w534 -> [w558]
              tunnel: w533 -> [w557]
              tunnel: w532 -> [w556]
              frame #0 {
                n127 = Wait (ms)(milliseconds to wait=w545) -> ()  [unwired: 1 out]
              }
              frame #1 {
                n128 = call-poly "Signals (Set).vi"("ISOBUS address"=w550, "error in"=w554, "PSU Act Stat"=T13 "CLMP", "Mercury Reference In"=w555) -> ("error out"=w552:errorcluster, "Mercury Reference Out"=w553:T11)  [unwired: 6 out]
              }
              frame #2 {
                n129 = Wait (ms)(milliseconds to wait=w556) -> ()  [unwired: 1 out]
              }
            }
          }
          event "Magnet Controls.TO SET": Mouse Down {
            n130 = event-data() -> ()  [unwired: 7 out]
            n131 = flat-sequence {
              tunnel: w567 -> [w575]
              tunnel: w572 -> [w576]
              tunnel: w573 -> [w577]
              tunnel: [w577] -> w566
              tunnel: [w576] -> w565
              tunnel: [w575] -> w564
              tunnel: [w574] -> w560
              tunnel: w559 -> [w574]
              tunnel: w566 -> [w584]
              tunnel: w565 -> [w583]
              tunnel: w564 -> [w579]
              tunnel: [w582] -> w563
              tunnel: [w581] -> w562
              tunnel: [w578] -> w561
              tunnel: w560 -> [w578]
              tunnel: [w586] -> w570
              tunnel: [w587] -> w571
              tunnel: w563 -> [w587]
              tunnel: w562 -> [w586]
              tunnel: w561 -> [w585]
              frame #0 {
                n132 = Wait (ms)(milliseconds to wait=w574) -> ()  [unwired: 1 out]
              }
              frame #1 {
                n133 = call-poly "Signals (Set).vi"("ISOBUS address"=w579, "error in"=w583, "PSU Act Stat"=T13 "RTOS", "Mercury Reference In"=w584) -> ("error out"=w581:errorcluster, "Mercury Reference Out"=w582:T11)  [unwired: 6 out]
              }
              frame #2 {
                n134 = Wait (ms)(milliseconds to wait=w585) -> ()  [unwired: 1 out]
              }
            }
          }
          event "Magnet Controls.TO ZERO": Mouse Down {
            n135 = event-data() -> ()  [unwired: 7 out]
            n136 = flat-sequence {
              tunnel: w596 -> [w604]
              tunnel: w601 -> [w605]
              tunnel: w602 -> [w606]
              tunnel: [w606] -> w595
              tunnel: [w605] -> w594
              tunnel: [w604] -> w593
              tunnel: [w603] -> w589
              tunnel: w588 -> [w603]
              tunnel: w595 -> [w613]
              tunnel: w594 -> [w612]
              tunnel: w593 -> [w608]
              tunnel: [w611] -> w592
              tunnel: [w610] -> w591
              tunnel: [w607] -> w590
              tunnel: w589 -> [w607]
              tunnel: [w615] -> w599
              tunnel: [w616] -> w600
              tunnel: w592 -> [w616]
              tunnel: w591 -> [w615]
              tunnel: w590 -> [w614]
              frame #0 {
                n137 = Wait (ms)(milliseconds to wait=w603) -> ()  [unwired: 1 out]
              }
              frame #1 {
                n138 = call-poly "Signals (Set).vi"("ISOBUS address"=w608, "error in"=w612, "PSU Act Stat"=T13 "RTOZ", "Mercury Reference In"=w613) -> ("error out"=w610:errorcluster, "Mercury Reference Out"=w611:T11)  [unwired: 6 out]
              }
              frame #2 {
                n139 = Wait (ms)(milliseconds to wait=w614) -> ()  [unwired: 1 out]
              }
            }
          }
          event "SWITCH\nHEATER": Mouse Down {
            n140 = event-data() -> ()  [unwired: 2 out]
            n141 = flat-sequence {
              tunnel: w637 -> [w646]
              tunnel: w638 -> [w647]
              tunnel: w639 -> [w648]
              tunnel: [w648] -> w620
              tunnel: [w647] -> w619
              tunnel: [w646] -> w618
              tunnel: w617 -> [w645]
              tunnel: [w654] -> w636
              tunnel: [w653] -> w635
              tunnel: [w650] -> w634
              tunnel: [w649] -> w628
              tunnel: w620 -> [w652]
              tunnel: w619 -> [w651]
              tunnel: w618 -> [w649]
              tunnel: w636 -> [w659]
              tunnel: w635 -> [w658]
              tunnel: w634 -> [w657]
              tunnel: [w659] -> w633
              tunnel: [w658] -> w632
              tunnel: [w657] -> w631
              tunnel: [w656] -> w629
              tunnel: w628 -> [w656]
              tunnel: w617 -> [w655]
              tunnel: w633 -> [w664]
              tunnel: w632 -> [w663]
              tunnel: w631 -> [w670]
              tunnel: w629 -> [w660]
              tunnel: [w665] -> w624
              tunnel: [w662] -> w623
              tunnel: [w661] -> w622
              tunnel: [w660] -> w621
              tunnel: [w672] -> w625
              tunnel: [w673] -> w626
              tunnel: [w674] -> w627
              tunnel: [w675] -> w630
              tunnel: w624 -> [w675]
              tunnel: w623 -> [w674]
              tunnel: w622 -> [w673]
              tunnel: w621 -> [w672]
              tunnel: w617 -> [w671]
              frame #0 {
                n142 = Wait (ms)(milliseconds to wait=w645) -> ()  [unwired: 1 out]
              }
              frame #1 {
                n143 = call-poly "Signals (Read).vi"("ISOBUS address"=w649, "error in"=w651, "Mercury Reference In"=w652) -> ("error out"=w653:errorcluster, "Current"=w650:dbl, "Mercury Reference Out"=w654:T11)  [unwired: 6 out]
              }
              frame #2 {
                n144 = Wait (ms)(milliseconds to wait=w655) -> ()  [unwired: 1 out]
              }
              frame #3 {
                n145 = call-poly "Signals (Read).vi"("ISOBUS address"=w660, "error in"=w663, "Mercury Reference In"=w664) -> ("error out"=w661:errorcluster, "Persistant Current"=w669:dbl, "Mercury Reference Out"=w662:T11)  [unwired: 6 out]
                n146 = Subtract(x=w669, y=w670) -> (x-y=w668:dbl)
                n147 = Absolute Value(x=w668) -> (abs(x)=w667:dbl)
                n148 = Less?(x=w667, y=0.1) -> (x < y?=w665:bool)
              }
              frame #4 {
                n149 = Wait (ms)(milliseconds to wait=w671) -> ()  [unwired: 1 out]
              }
            }
            n150 = case shown="False" w630 {
              selector: w630 -> [_ w678]
              tunnel: [w677 w678] -> w640
              frame False {
                n151 = Two Button Dialog(message="The magnet current is more\nthan 0.1A different to the\nPSU output current.  It is not\nadvisable to switch on the\nswitch heater unless these\ncurrents are equal!") -> (T button?=w677:bool)  [unwired: 2 out]
              }
              frame True {
              }
            }
            n152 = case shown="True" w640 {
              tunnel: w627 -> [w680 w697]
              tunnel: w626 -> [w679 w696]
              tunnel: [w680 w695] -> w642
              tunnel: [w679 w694] -> w641
              tunnel: w625 -> [_ w693]
              tunnel: w617 -> [_ w682]
              tunnel: w617 -> [_ w681]
              frame False {
              }
              frame True {
                n153 = flat-sequence {
                  tunnel: [w707] -> w703
                  tunnel: [w706] -> w702
                  tunnel: [w705] -> w701
                  tunnel: w697 -> [w709]
                  tunnel: w696 -> [w708]
                  tunnel: w693 -> [w704]
                  tunnel: [w704] -> w691
                  tunnel: w703 -> [w713]
                  tunnel: w702 -> [w712]
                  tunnel: [w713] -> w700
                  tunnel: [w712] -> w699
                  tunnel: [w711] -> w698
                  tunnel: w701 -> [w711]
                  tunnel: [w710] -> w692
                  tunnel: w691 -> [w710]
                  tunnel: w700 -> [w724]
                  tunnel: w699 -> [w725]
                  tunnel: w698 -> [w722]
                  tunnel: [w719] -> w688
                  tunnel: [w720] -> w686
                  tunnel: w692 -> [w715]
                  tunnel: [w715] -> w684
                  tunnel: w688 -> [w729]
                  tunnel: [w729] -> w687
                  tunnel: w686 -> [w728]
                  tunnel: [w728] -> w685
                  tunnel: w684 -> [w727]
                  tunnel: [w727] -> w683
                  tunnel: w682 -> [w726]
                  tunnel: w687 -> [w735]
                  tunnel: w685 -> [w734]
                  tunnel: w683 -> [w730]
                  tunnel: [w733] -> w690
                  tunnel: [w732] -> w689
                  tunnel: [w737] -> w694
                  tunnel: [w738] -> w695
                  tunnel: w690 -> [w738]
                  tunnel: w689 -> [w737]
                  tunnel: w681 -> [w736]
                  frame #0 {
                    n154 = call-poly "Signals (Read).vi"("ISOBUS address"=w704, "error in"=w708, "Mercury Reference In"=w709) -> ("error out"=w707:errorcluster, "Switch Heater Status"=w705:string, "Mercury Reference Out"=w706:T11)  [unwired: 6 out]
                  }
                  frame #1 {
                    n155 = Wait Until Next ms Multiple(millisecond multiple=u32 100) -> ()  [unwired: 1 out]
                  }
                  frame #2 {
                    n156 = Equal?(x=w722, y="ON") -> (x = y?=w721:bool)
                    n157 = Select(t=T14 "OFF" ("Set Switch Heater"), s=w721, f=T14 "ON" ("Set Switch Heater")) -> (s? t:f=w716:T14)
                    n158 = call-poly "Signals (Set).vi"("ISOBUS address"=w715, "error in"=w724, "Set Switch Heater"=w716, "Mercury Reference In"=w725) -> ("error out"=w720:errorcluster, "Mercury Reference Out"=w719:T11)  [unwired: 6 out]
                  }
                  frame #3 {
                    n159 = Wait (ms)(milliseconds to wait=w726) -> ()  [unwired: 1 out]
                  }
                  frame #4 {
                    n160 = call-poly "Configuration (Read).vi"("ISOBUS address"=w730, "error in"=w734, "Mercury Reference In"=w735) -> ("error out"=w732:errorcluster, "time stamp"=→"Switch TS":timestamp, "Mercury Reference Out"=w733:T11)  [unwired: 6 out]
                  }
                  frame #5 {
                    n161 = Wait (ms)(milliseconds to wait=w736) -> ()  [unwired: 1 out]
                  }
                }
              }
            }
          }
          event "Ramp Controls": Value Change {
            n162 = event-data() -> ()  [unwired: 6 out]
            n163 = case shown="True" w748 {
              tunnel: w754 -> [w783 w842]
              tunnel: w753 -> [w782 w841]
              tunnel: [w770 w826] -> w752
              tunnel: [w769 w825] -> w751
              tunnel: w747 -> [w759 _]
              tunnel: w746 -> [w760 _]
              tunnel: w745 -> [_ w811]
              tunnel: w744 -> [_ w812]
              tunnel: w743 -> [w771 w840]
              tunnel: w742 -> [w762 w817]
              tunnel: w741 -> [w756 w814]
              tunnel: w740 -> [w758 w813]
              tunnel: [w755 w810] -> w739
              frame False {
                n164 = Divide(x=w760, y=w758) -> (x/y=w761:dbl)
                n165 = Divide(x=w759, y=w758) -> (x/y=w757:dbl)
                n166 = Bundle By Name(cluster=w756, "Target Field (T)"=w761, "Target Rate (T/min)"=w757) -> (w755:T8)
                n167 = flat-sequence {
                  tunnel: w760 -> [w786]
                  tunnel: w782 -> [w787]
                  tunnel: w783 -> [w788]
                  tunnel: [w788] -> w781
                  tunnel: [w787] -> w780
                  tunnel: [w786] -> w779
                  tunnel: [w785] -> w772
                  tunnel: w771 -> [w785]
                  tunnel: [w784] -> w763
                  tunnel: w762 -> [w784]
                  tunnel: w781 -> [w795]
                  tunnel: w780 -> [w794]
                  tunnel: w779 -> [w791]
                  tunnel: [w793] -> w778
                  tunnel: [w792] -> w777
                  tunnel: [w790] -> w773
                  tunnel: w772 -> [w790]
                  tunnel: [w789] -> w764
                  tunnel: w763 -> [w789]
                  tunnel: w778 -> [w799]
                  tunnel: w777 -> [w798]
                  tunnel: [w799] -> w776
                  tunnel: [w798] -> w775
                  tunnel: [w797] -> w774
                  tunnel: w773 -> [w797]
                  tunnel: [w796] -> w765
                  tunnel: w764 -> [w796]
                  tunnel: w776 -> [w806]
                  tunnel: w775 -> [w805]
                  tunnel: w759 -> [w804]
                  tunnel: w774 -> [w801]
                  tunnel: [w803] -> w768
                  tunnel: [w802] -> w767
                  tunnel: [w800] -> w766
                  tunnel: w765 -> [w800]
                  tunnel: [w808] -> w769
                  tunnel: [w809] -> w770
                  tunnel: w768 -> [w809]
                  tunnel: w767 -> [w808]
                  tunnel: w766 -> [w807]
                  frame #0 {
                    n168 = Wait (ms)(milliseconds to wait=w784) -> ()  [unwired: 1 out]
                  }
                  frame #1 {
                    n169 = call-poly "Signals (Set).vi"("ISOBUS address"=w790, "error in"=w794, "Target Current"=w791, "Mercury Reference In"=w795) -> ("error out"=w792:errorcluster, "Mercury Reference Out"=w793:T11)  [unwired: 1 in, 5 out]
                  }
                  frame #2 {
                    n170 = Wait (ms)(milliseconds to wait=w796) -> ()  [unwired: 1 out]
                  }
                  frame #3 {
                    n171 = call-poly "Signals (Set).vi"("ISOBUS address"=w801, "error in"=w805, "Target Current Rate"=w804, "Mercury Reference In"=w806) -> ("error out"=w802:errorcluster, "Mercury Reference Out"=w803:T11)  [unwired: 1 in, 5 out]
                  }
                  frame #4 {
                    n172 = Wait (ms)(milliseconds to wait=w807) -> ()  [unwired: 1 out]
                  }
                }
              }
              frame True {
                n173 = Multiply(x=w812, y=w813) -> (x*y=w816:dbl)
                n174 = Multiply(x=w811, y=w813) -> (x*y=w815:dbl)
                n175 = flat-sequence {
                  tunnel: w811 -> [w844]
                  tunnel: w840 -> [w845]
                  tunnel: w812 -> [w846]
                  tunnel: w841 -> [w847]
                  tunnel: w842 -> [w848]
                  tunnel: [w848] -> w839
                  tunnel: [w847] -> w838
                  tunnel: [w846] -> w837
                  tunnel: [w845] -> w836
                  tunnel: [w844] -> w835
                  tunnel: [w843] -> w818
                  tunnel: w817 -> [w843]
                  tunnel: w839 -> [w856]
                  tunnel: w838 -> [w855]
                  tunnel: w837 -> [w852]
                  tunnel: w836 -> [w851]
                  tunnel: w835 -> [w850]
                  tunnel: [w854] -> w834
                  tunnel: [w853] -> w833
                  tunnel: [w851] -> w832
                  tunnel: [w850] -> w831
                  tunnel: [w849] -> w819
                  tunnel: w818 -> [w849]
                  tunnel: w834 -> [w861]
                  tunnel: w833 -> [w860]
                  tunnel: w832 -> [w859]
                  tunnel: w831 -> [w858]
                  tunnel: [w861] -> w830
                  tunnel: [w860] -> w829
                  tunnel: [w859] -> w828
                  tunnel: [w858] -> w827
                  tunnel: [w857] -> w820
                  tunnel: w819 -> [w857]
                  tunnel: w830 -> [w868]
                  tunnel: w829 -> [w867]
                  tunnel: w828 -> [w865]
                  tunnel: w827 -> [w866]
                  tunnel: [w865] -> w824
                  tunnel: [w864] -> w823
                  tunnel: [w863] -> w822
                  tunnel: [w862] -> w821
                  tunnel: w820 -> [w862]
                  tunnel: [w870] -> w826
                  tunnel: [w871] -> w825
                  tunnel: [w872] -> _
                  tunnel: w824 -> [w872]
                  tunnel: w823 -> [w871]
                  tunnel: w822 -> [w870]
                  tunnel: w821 -> [w869]
                  frame #0 {
                    n176 = Wait (ms)(milliseconds to wait=w843) -> ()  [unwired: 1 out]
                  }
                  frame #1 {
                    n177 = call-poly "Signals (Set).vi"("ISOBUS address"=w851, "error in"=w855, "Target Field"=w852, "Mercury Reference In"=w856) -> ("error out"=w853:errorcluster, "Mercury Reference Out"=w854:T11)  [unwired: 1 in, 5 out]
                  }
                  frame #2 {
                    n178 = Wait (ms)(milliseconds to wait=w857) -> ()  [unwired: 1 out]
                  }
                  frame #3 {
                    n179 = call-poly "Signals (Set).vi"("ISOBUS address"=w865, "error in"=w867, "Target Field Rate"=w866, "Mercury Reference In"=w868) -> ("error out"=w864:errorcluster, "Mercury Reference Out"=w863:T11)  [unwired: 1 in, 5 out]
                  }
                  frame #4 {
                    n180 = Wait (ms)(milliseconds to wait=w869) -> ()  [unwired: 1 out]
                  }
                }
                n181 = Bundle By Name(cluster=w814, "Target Current (A)"=w816, "Target Rate (A/min)"=w815) -> (w810:T8)
              }
            }
            n182 = local write "Ramp Controls"(w739) -> ()
          }
          event "stop": Mouse Down {
            n183 = event-data() -> ()  [unwired: 2 out]
          }
          event "Display Units": Value Change {
            n184 = event-data() -> ()  [unwired: 6 out]
            n185 = property on="Output (T) (Field equivalent)" class="DigNum (strict)"(error in=w888, "Visible"=w879) -> (error out=w887:errorcluster)  [unwired: 1 in, 1 out]
            n186 = property on="Magnet Centre Field (T)" class="DigNum (strict)"(error in=w887, "Visible"=w879) -> (error out=w886:errorcluster)  [unwired: 1 in, 1 out]
            n187 = property on="Target Rate (T/min)" class="DigNum (strict)"(error in=w886, "Visible"=w879) -> (error out=w885:errorcluster)  [unwired: 1 in, 1 out]
            n188 = property on="Target Field (T)" class="DigNum (strict)"(error in=w885, "Visible"=w879) -> (error out=w884:errorcluster)  [unwired: 1 in, 1 out]
            n189 = Not(x=w879) -> (.not. x?=w878:bool)
            n190 = property on="Output Current (A)" class="DigNum (strict)"(error in=w884, "Visible"=w878) -> (error out=w883:errorcluster)  [unwired: 1 in, 1 out]
            n191 = property on="Magnet Current (A)" class="DigNum (strict)"(error in=w883, "Visible"=w878) -> (error out=w882:errorcluster)  [unwired: 1 in, 1 out]
            n192 = property on="Target Current (A)" class="DigNum (strict)"(error in=w882, "Visible"=w878) -> (error out=w881:errorcluster)  [unwired: 1 in, 1 out]
            n193 = property on="Target Rate (A/min)" class="DigNum (strict)"(error in=w881, "Visible"=w878) -> (error out=w880:errorcluster)  [unwired: 1 in, 1 out]
          }
        }
        n194 = Wait Until Next ms Multiple(millisecond multiple=u32 1000) -> ()  [unwired: 1 out]
      }
      n195 = property on="Current (A)" class="Knob (strict)"("Scale.Minimum"=w159, "Scale.Maximum"=w158) -> ()  [unwired: 2 in, 2 out]
      n196 = property on="Voltage (V)" class="Knob (strict)"("Scale.Minimum"=w157, "Scale.Maximum"=w156) -> ()  [unwired: 2 in, 2 out]
    }
  }
  n197 = call "Close.vi"("error in (no error)"=w43, "Mercury Reference"=w44) -> ("error out"=→"error out":errorcluster)  [unwired: 9 out]
  "Sys_time_stamp" <- w1
